vi "SubVI TX Awgn channel.vi"(2 "噪声功率(dB)":dbl, 8 "错误输入":errorcluster, 11 "输入":cdb[](array[numeric])) -> (0 "错误输出":errorcluster, 3 "输出":cdb[](array[numeric]))   [LabVIEW 2015]
uses:
  <vilib>/Analysis/NI_AALBase.lvlib
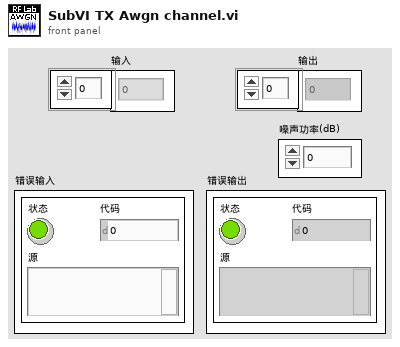
[diagram p1: front panel]
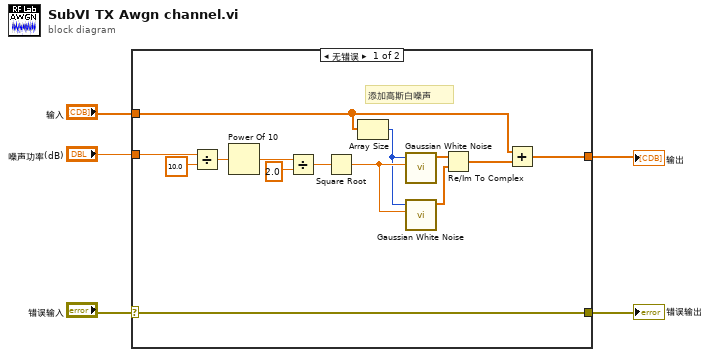
[diagram p0: block diagram]
diagram:
  n1 = case shown="无错误" "错误输入" {
    selector: "错误输入" -> [w9 w20]
    tunnel: [w9 w20] -> w2
    tunnel: "噪声功率(dB)" -> [w8 _]
    tunnel: "输入" -> [w7 _]
    tunnel: [w6 _] -> w5
    frame No Error {
      # "添加高斯白噪声"
      n2 = Divide(x=w8, y=10.0) -> (x/y=w19:dbl)
      n3 = Power Of 10(x=w19) -> (10^x=w15:dbl)
      n4 = Divide(x=w15, y=2.0) -> (x/y=w16:dbl)
      n5 = Square Root(x=w16) -> (sqrt(x)=w14:dbl)
      n6 = Array Size(array=w7) -> (size(s)=w13:i32)
      n7 = call <vilib>:"Gaussian White Noise.vi"("standard deviation"=w14, "samples"=w13) -> ("Gaussian noise pattern"=w10:dbl[])  [unwired: 8 in, 1 out]
      n8 = call <vilib>:"Gaussian White Noise.vi"("standard deviation"=w14, "samples"=w13) -> ("Gaussian noise pattern"=w11:dbl[])  [unwired: 8 in, 1 out]
      n9 = Re/Im To Complex(1:w11, 2:w10) -> (0:w12:cdb[])
      n10 = Add(x=w7, y=w12) -> (x+y=w6:cdb[])
    }
    frame Error {
    }
  }
  "输出" <- w5
  "错误输出" <- w2
